vi "ForLoop.vi"() -> ()   [LabVIEW 2020]
panel:
  out "x+y":dbl
  out "Numeric 2":i32
  in  "Numeric":i32
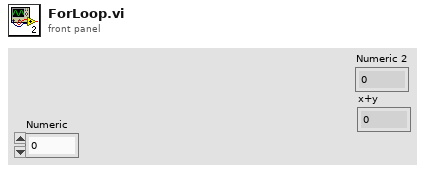
[diagram p1: front panel]
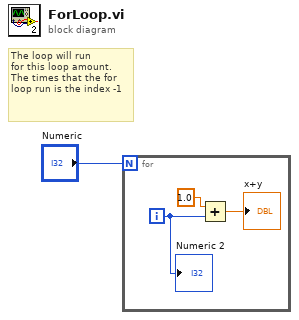
[diagram p0: block diagram]
diagram:
  # "The loop will run\nfor this loop amount. The times that the for loop run is the index -1"
  n1 = for {
    N: "Numeric" -> [_]
    i -> [w3]
    n2 = Add(x=1.0, y=w3) -> (x+y=→"x+y":dbl)
    "Numeric 2" <- w3
  }
